vi "HotButton.vi"(11 "Buttons[0]":bool) -> (3 "Boolean":bool)   [LabVIEW 2017]
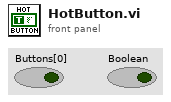
[diagram p1: front panel]
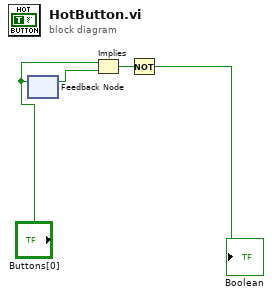
[diagram p0: block diagram]
diagram:
  n1 = feedback #1() -> (w3:bool)  [unwired: 1 in]
  n2 = feedback-in #1("Buttons[0]") -> ()
  n3 = Implies(1:w3, 2:"Buttons[0]") -> (0:w1:bool)
  n4 = Not(x=w1) -> (.not. x?=→"Boolean":bool)
